vi "PH_Beckhoff_StepMot.declare digital OutputTags.vi"(3 "Instance Name":string="N/A") -> (0 "Digital Outputs":T1, 1 "Description":string)   [LabVIEW 2014, in "PH_Beckhoff_StepMot.lvlib"]
uses:
  PH_Beckhoff_StepMot.lvlib
  PH_Beckhoff/PH_Beckhoff.Digital Outputs.ctl
  PH_Beckhoff/PH_Beckhoff.lvlib
panel:
  out "Right Size?":bool
  # "Let this VI run to check the size!"
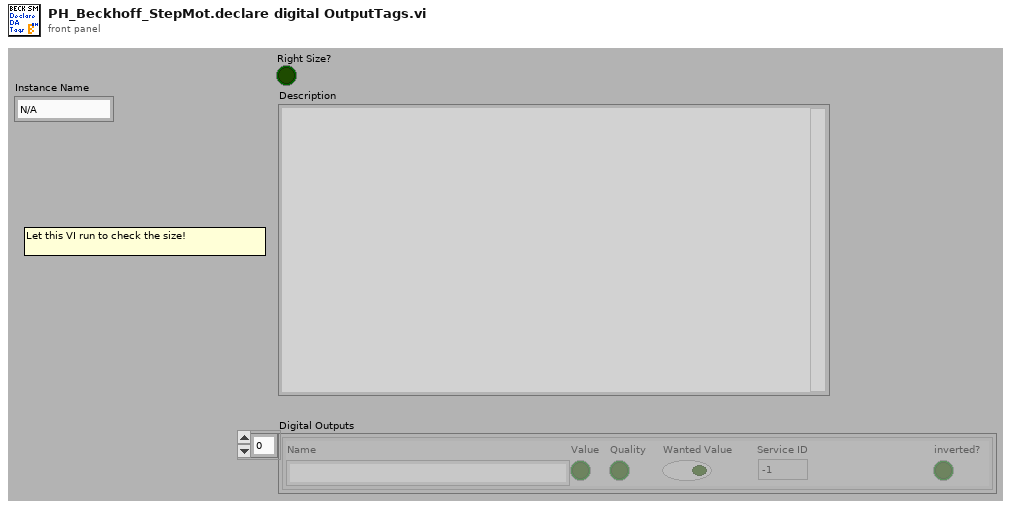
[diagram p1: front panel]
types:
  T1 = typedef "PH_Beckhoff.lvlib/PH_Beckhoff.Digital Outputs.ctl" = cluster{"Name":string, "Value":bool, "Quality":bool, "Wanted Value":bool, "Service ID":i32, "inverted?":bool}[]
  T2 = cluster{"Name":string, "Value":bool, "Quality":bool, "Wanted Value":bool, "Service ID":i32, "inverted?":bool}
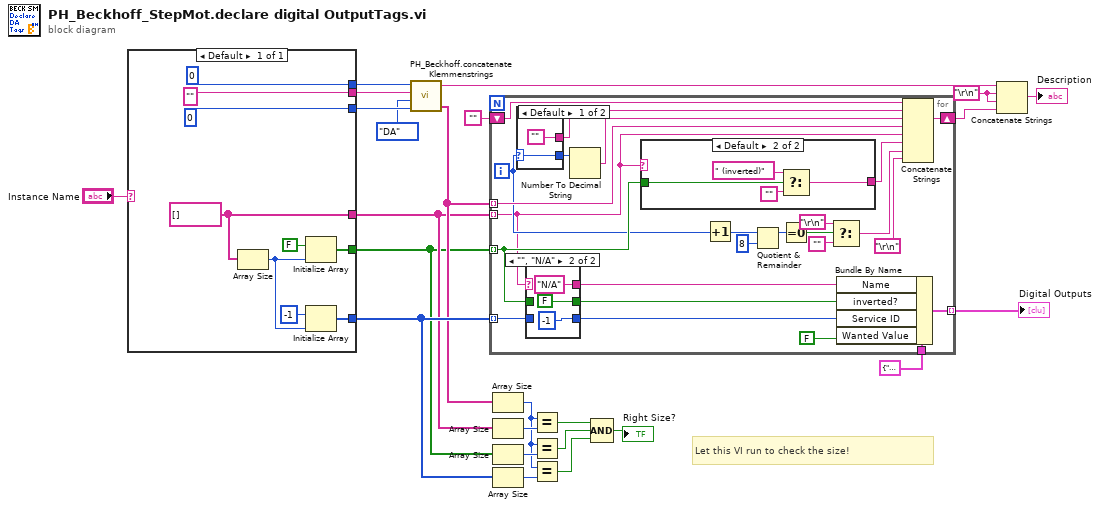
[diagram p0: block diagram]
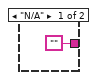
[diagram p2: hidden frame]
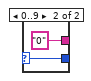
[diagram p4: hidden frame]
diagram:
  w22 = "\r\n"
  # "Let this VI run to check the size!"
  n1 = case shown="Default" "Instance Name" {
    tunnel: [0 ("size(s)")] -> w21
    tunnel: ["" ("Klemmenname")] -> w20
    tunnel: [0 ("# of In- or Outputs")] -> w9
    tunnel: [w29] -> w7
    tunnel: [w28] -> w3
    tunnel: [w25] -> w2
    frame Default {
      w28 = string[] [] ("appended array")
      n2 = Array Size(array=w28) -> (size(s)=w26:i32)
      n3 = Initialize Array(FALSE, w26) -> (w25:bool[])
      n4 = Initialize Array(-1 ("Service ID"), w26) -> (w29:i32[])
    }
  }
  n5 = call "PH_Beckhoff.concatenate Klemmenstrings.vi"("# of In- or Outputs"=w9, "Type"=enum16{"AE", "AA", "DE", "DA", "SE"}."DA", "Klemmenname"=w20, "Quantity"=w21) -> ("concatenated string array"=w5:string[], "\"<Type>: <Quantity> x <Klemmenname>\""=w4:string)  [unwired: 1 out]
  n6 = for {
    tunnel: w3 -> [w37] mode=indexing
    tunnel: w5 -> [w46] mode=indexing
    shift-right: [w49] -> w23
    shift-left: "" -> [w50]
    tunnel: T2 {"Name"="", "Value"=FALSE, "Quality"=FALSE, "Wanted Value"=FALSE, "Service ID"=0, "inverted?"=FALSE} ("Digital Input Value") -> [w36]
    tunnel: [w55] -> w18 mode=indexing
    tunnel: w2 -> [w51] mode=indexing
    tunnel: w7 -> [w54] mode=indexing
    i -> [w39]
    n7 = case shown="Default" w39 {
      selector: w39 -> [w70 w73]
      tunnel: [w70 w73] -> w58
      tunnel: ["" "0"] -> w57
      frame Default {
      }
      frame 0..9 {
      }
    }
    n8 = case shown="\"\", \"N/A\"" w37 {
      selector: w37 -> [w64 _]
      tunnel: w54 -> [w66 _]
      tunnel: [w66 -1 ("Service ID")] -> w53
      tunnel: w51 -> [w65 _]
      tunnel: [w65 FALSE ("element")] -> w52
      tunnel: [w64 "N/A"] -> w35
      frame Default {
      }
      frame "", "N/A" {
      }
    }
    n9 = Number To Decimal String(number=w58) -> (decimal integer string=w56:string)  [unwired: 1 in]
    n10 = case shown="Default" w37 {
      tunnel: w51 -> [_ w63]
      tunnel: ["" w60] -> w48
      frame "N/A" {
      }
      frame Default {
        n11 = Select(t=" (inverted)" ("string"), s=w63, f="") -> (s? t:f=w60:string)
      }
    }
    n12 = Increment(x=w39) -> (x+1=w41:i32)
    n13 = Quotient & Remainder(x=w41, y=8) -> (x-y*floor(x/y)=w43:i32)  [unwired: 1 out]
    n14 = Equal To 0?(x=w43) -> (x = 0?=w44:bool)
    n15 = Select(t="\r\n", s=w44, f="") -> (s? t:f=w40:string)
    n16 = Bundle By Name(cluster=w36, "Name"=w35, "inverted?"=w52, "Service ID"=w53, "Wanted Value"=FALSE) -> (w55:T2)
    n17 = Concatenate Strings(w50, w57, w56, w46, w37, w48, w40, "\r\n") -> (w49:string)
  }
  "Digital Outputs" <- w18
  n18 = Array Size(array=w5) -> (size(s)=w11:i32)
  n19 = Array Size(array=w3) -> (size(s)=w13:i32)
  n20 = Array Size(array=w2) -> (size(s)=w12:i32)
  n21 = Array Size(array=w7) -> (size(s)=w17:i32)
  n22 = Equal?(x=w11, y=w13) -> (x = y?=w16:bool)
  n23 = Equal?(x=w11, y=w12) -> (x = y?=w10:bool)
  n24 = Equal?(x=w11, y=w17) -> (x = y?=w15:bool)
  n25 = Compound Arithmetic op=AND(w16, w10, w15) -> (→"Right Size?":bool)
  n26 = Concatenate Strings(w4, w22, w22, w23) -> (→"Description":string)
